vi "Generate Simulated Data.vi"(6 "Acquisition":refnum<queue>, 7 "Bits":bool[][](array[boolean]), 8 "error in (no error)":errorcluster, 10 "Longueur d'onde":dbl, 11 "Loop Count":dbl) -> (0 "error out":errorcluster, 2 "Data Out":variant[](array[variant]), 3 "Disconnected":bool=TRUE)   [LabVIEW 2018, in "Acquisition.lvlib"]
doc: "Generates sample waveforms according to the signal type in the HW Config input."
uses:
  Acquisition.lvlib
  GlobalVariable/GlobalPowerByTime.vi
  GlobalVariable/Globalt0.vi
  support/Message Queue/Message Queue.lvlib
  <vilib>/gmath/NI_Gmath.lvlib
  GlobalVariable/GlobalSet0.vi
  <vilib>/Analysis/NI_AALPro.lvlib
  GlobalVariable/GlobalPosXbyTime.vi
  GlobalVariable/GlobalPosYbyTime.vi
  GlobalVariable/GlobalProfileByTime.vi
  GlobalVariable/GlobalTimeStep.vi
  GlobalVariable/GlobalTensionByTime.vi
  GlobalVariable/GlobalTemperatureByTime.vi
  support/Message Queue/Enqueue Message (Single).vi
  <vilib>/gmath/interp.llb/Create Mesh Grid (2D) (x,y arrays).vi
  <vilib>/Analysis/2dsp.llb/2D Convolution (DBL).vi
  <vilib>/DAQmx/create/channels.llb/DAQmx Create Channel (DO-Digital Output).vi
  <resource>/objmgr/daqmx.rc
  <vilib>/Analysis/NI_AALBase.lvlib
  <vilib>/Analysis/baseanly.llb/Mean (DBL).vi
  <vilib>/DAQmx/create/channels.llb/DAQmx Create Channel (AI-Voltage-Basic).vi
  <vilib>/DAQmx/configure/timing.llb/DAQmx Timing (Sample Clock).vi
  <vilib>/DAQmx/read.llb/DAQmx Read (Analog 1D Wfm NChan NSamp).vi
  <vilib>/DAQmx/write.llb/DAQmx Write (Digital 1D Bool NChan 1Samp 1Line).vi
  support/Message Queue/Message Cluster.ctl
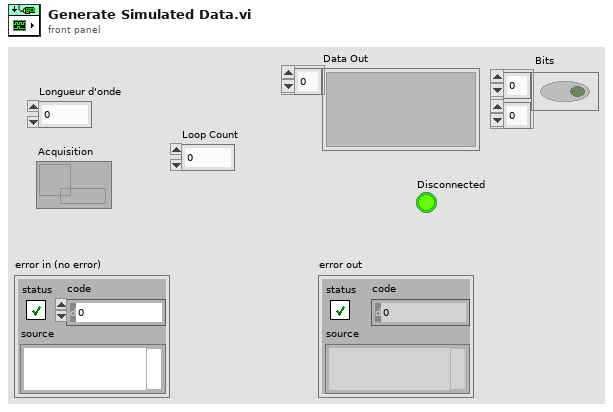
[diagram p1: front panel]
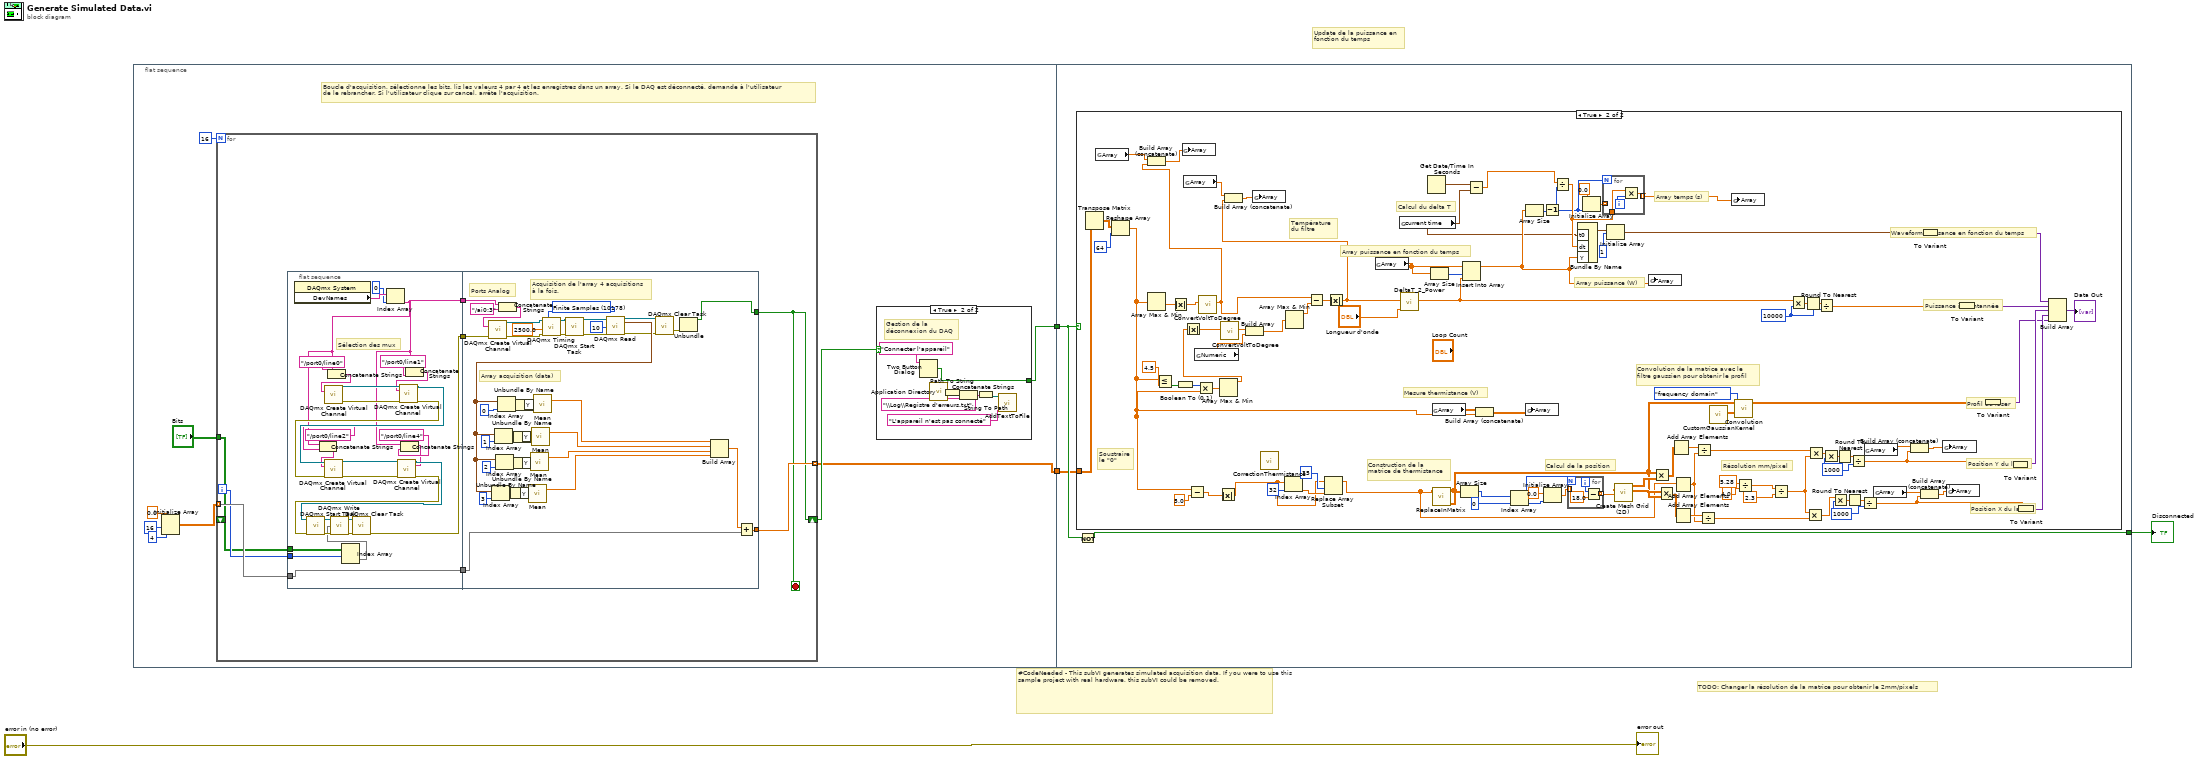
[diagram p0: block diagram]
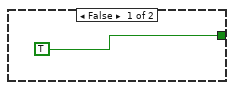
[diagram p2: hidden frame]
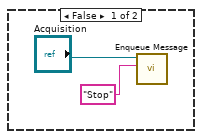
[diagram p3: hidden frame]
diagram:
  # "TODO: Changer la résolution de la matrice pour obtenir le 2mm/pixels"
  # "Update de la puissance en\nfonction du temps"
  # "#CodeNeeded - This subVI generates simulated acquisition data. If you were to use this sample project with real hardware, this subVI could be removed."
  n1 = flat-sequence {
    tunnel: [w8] -> w3
    tunnel: [w6] -> w1
    tunnel: w3 -> [w98]
    tunnel: [w97] -> w2
    tunnel: w1 -> [w96]
    frame #0 {
      # "Boucle d'acquisition, sélectionne les bits, lis les valeurs 4 par 4 et les enregistres dans un array. Si le DAQ est déconnecté, demande à l'utilisateur \nde le rebrancher. Si l'utilisateur clique sur cancel, arrête l'acquisition."
      n2 = Initialize Array(0.0 ("element"), 16 ("dimension size"), 4 ("dimension size")) -> (w9:dbl[][])
      n3 = for {
        N: 16 -> [_]
        tunnel: "Bits" -> [w25]
        tunnel: w9 -> [w30] mode=indexing
        tunnel: [w24] -> w6 mode=indexing
        shift-right: [w23] -> w7
        shift-left: _ -> [_]
        i -> [w26]
        stop <- w23 stop-if-true
        n4 = flat-sequence {
          tunnel: w26 -> [w44]
          tunnel: [w55] -> w29
          tunnel: w25 -> [w43]
          tunnel: [w31] -> w28
          tunnel: [w32] -> w27
          tunnel: w30 -> [w31]
          tunnel: w29 -> [w87]
          tunnel: w28 -> [w67]
          tunnel: [w69] -> w24
          tunnel: w27 -> [w64]
          tunnel: [w59] -> w23
          frame #0 {
            # "Sélection des mux"
            n5 = property class="DAQmx System"() -> ("DevNames"=w42:tag[])  [unwired: 2 in, 2 out]
            n6 = Index Array(array=w43, index (row)=w44) -> (element=w56:bool[])  [unwired: 1 in]
            n7 = Index Array(array=w42, index=0) -> (element=w32:tag)
            n8 = Concatenate Strings(w32, "/port0/line2" ("string")) -> (w35:string)
            n9 = Concatenate Strings(w32, "/port0/line0" ("string")) -> (w40:string)
            n10 = call-poly <vilib>:"DAQmx Create Virtual Channel.vi"("lines"=w40) -> ("task out"=w51:refnum<k21>, "error out"=w52:errorcluster)  [unwired: 13 in]
            n11 = Concatenate Strings(w32, "/port0/line4" ("string")) -> (w33:string)
            n12 = Concatenate Strings(w32, "/port0/line1" ("string")) -> (w37:string)
            n13 = call-poly <vilib>:"DAQmx Create Virtual Channel.vi"("task in"=w51, "lines"=w37, "error in"=w52) -> ("task out"=w50:refnum<k21>, "error out"=w49:errorcluster)  [unwired: 11 in]
            n14 = call-poly <vilib>:"DAQmx Create Virtual Channel.vi"("task in"=w50, "lines"=w35, "error in"=w49) -> ("task out"=w47:refnum<k21>, "error out"=w48:errorcluster)  [unwired: 11 in]
            n15 = call-poly <vilib>:"DAQmx Create Virtual Channel.vi"("task in"=w47, "lines"=w33, "error in"=w48) -> ("task out"=w46:refnum<k21>, "error out"=w45:errorcluster)  [unwired: 11 in]
            n16 = call <vilib>:"DAQmx Start Task.vi"("task/channels in"=w46, "error in"=w45) -> ("task out"=w57:refnum<k21>, "error out"=w58:errorcluster)  [unwired: 12 in]
            n17 = call-poly <vilib>:"DAQmx Write.vi"("task/channels in"=w57, "data"=w56, "error in"=w58) -> ("task out"=w54:refnum<k21>, "error out"=w53:errorcluster)  [unwired: 10 in, 1 out]
            n18 = call <vilib>:"DAQmx Clear Task.vi"("task in"=w54, "error in"=w53) -> ("error out"=w55:errorcluster)  [unwired: 13 in]
          }
          frame #1 {
            w89 = 10178 items=["Finite Samples"=10178, "Continuous Samples"=10123, "Hardware Timed Single Point"=12522] ("sample mode")
            # "Ports Analog"
            # "Array acquisition (data)"
            # "Acquisition de l'array 4 acquisitions\nà la fois."
            n19 = Concatenate Strings(w64, "/ai0:3" ("string")) -> (w65:string)
            n20 = call-poly <vilib>:"DAQmx Create Virtual Channel.vi"("physical channels"=w65, "error in"=w87) -> ("task out"=w94:refnum<k21>, "error out"=w93:errorcluster)  [unwired: 12 in]
            n21 = call-poly <vilib>:"DAQmx Timing.vi"("task/channels in"=w94, "sample mode"=w89, "rate"=2500.0, "error in"=w93) -> ("task out"=w90:refnum<k21>, "error out"=w91:errorcluster)  [unwired: 10 in]
            n22 = call <vilib>:"DAQmx Start Task.vi"("task/channels in"=w90, "error in"=w91) -> ("task out"=w92:refnum<k21>, "error out"=w95:errorcluster)  [unwired: 12 in]
            n23 = call-poly <vilib>:"DAQmx Read.vi"("task/channels in"=w92, "number of samples per channel"=10, "error in"=w95) -> ("task out"=w71:refnum<k21>, "data"=w80:waveform(dbl)[], "error out"=w70:errorcluster)  [unwired: 10 in]
            n24 = Index Array(array=w80, index=3) -> (element=w76:waveform(dbl))
            n25 = Index Array(array=w80, index=1) -> (element=w78:waveform(dbl))
            n26 = Index Array(array=w80, index=2) -> (element=w77:waveform(dbl))
            n27 = Index Array(array=w80, index=0) -> (element=w79:waveform(dbl))
            n28 = Unbundle By Name(w76) -> ("Y"=w72:dbl[])
            n29 = Unbundle By Name(w78) -> ("Y"=w74:dbl[])
            n30 = Unbundle By Name(w77) -> ("Y"=w73:dbl[])
            n31 = Unbundle By Name(w79) -> ("Y"=w75:dbl[])
            n32 = call-poly <vilib>:"Mean.vi"("X"=w72) -> ("mean"=w60:dbl)  [unwired: 1 out]
            n33 = call-poly <vilib>:"Mean.vi"("X"=w73) -> ("mean"=w61:dbl)  [unwired: 1 out]
            n34 = call-poly <vilib>:"Mean.vi"("X"=w74) -> ("mean"=w62:dbl)  [unwired: 1 out]
            n35 = call-poly <vilib>:"Mean.vi"("X"=w75) -> ("mean"=w63:dbl)  [unwired: 1 out]
            n36 = call <vilib>:"DAQmx Clear Task.vi"("task in"=w71, "error in"=w70) -> ("error out"=w85:errorcluster)  [unwired: 13 in]
            n37 = Unbundle(w85) -> ("status"=w59:bool)  [unwired: 2 out]
            n38 = Build Array(w63, w62, w61, w60) -> (w68:dbl[])
            n39 = Add(x=w68, y=w67) -> (x+y=w69:dbl[])
          }
        }
      }
      n40 = case shown="True" w7 {
        tunnel: [TRUE w22] -> w8
        frame False {
        }
        frame True {
          # "Gestion de la \ndéconnexion du DAQ"
          n41 = Two Button Dialog(message="Connecter l'appareil") -> (T button?=w22:bool)  [unwired: 2 in]
          n42 = call <vilib>:"Application Directory.vi"() -> ("Application Directory"=w19:path)
          n43 = Path To String(path=w19) -> (string=w20:string)
          n44 = Concatenate Strings(w20, "\\Log\\Registre d'erreurs.txt") -> (w21:string)
          n45 = String To Path(string=w21) -> (path=w15:path)
          n46 = call "AddTextToFile.vi"("Ajouter du texte"="L'appareil n'est pas connecté", "Fichier"=w15) -> ()  [unwired: 10 in]
        }
      }
    }
    frame #1 {
      n47 = case shown="True" w98 {
        tunnel: w96 -> [_ w101]
        frame False {
          n48 = call-poly "Enqueue Message.vi"("Message"="Stop", "Message Queue"="Acquisition") -> ()  [unwired: 8 in, 2 out]
        }
        frame True {
          w157 = 1000
          w161 = 1000
          w167 = 10000
          # "Résolution mm/pixel"
          # "Calcul du delta T"
          # "Mesure thermistance (V)"
          # "Soustraire\nle \"0\""
          # "Température \ndu filtre"
          # "Calcul de la position"
          # "Construction de la \nmatrice de thermistance"
          # "Position X du laser"
          # "Position Y du laser"
          # "Profil du laser"
          # "Puissance instantannée"
          # "Waveform puissance en fonction du temps"
          # "Array puissance (W)"
          # "Array temps (s)"
          # "Convolution de la matrice avec le \nfiltre gaussien pour obtenir le profil"
          # "Array puissance en fonction du temps"
          n49 = Transpose Matrix(1:w101) -> (0:w104:dbl[][])
          n50 = global read "GlobalTensionByTime.vi" "Array"() -> (w137:dbl[])
          n51 = Reshape Array(w104, 64 ("dimension size")) -> (w102:dbl[])
          n52 = Array Max & Min(array=w102) -> (min value=w130:dbl)  [unwired: 3 out]
          n53 = Less Or Equal?(x=w102, y=4.5) -> (x <= y?=w122:bool[])
          n54 = Absolute Value(x=w130) -> (abs(x)=w126:dbl)
          n55 = Boolean To (0,1)(Boolean=w122) -> (0, 1=w121:i16[])
          n56 = global read "GlobalTemperatureByTime.vi" "Array"() -> (w134:dbl[])
          n57 = Subtract(x=w102, y=5.0) -> (x-y=w124:dbl[])
          n58 = global read "GlobalSet0.vi" "Numeric"() -> (w108:dbl)
          n59 = Multiply(x=w121, y=w102) -> (x*y=w120:dbl[])
          n60 = call "ConvertVoltToDegree.vi"("Tension"=w126) -> ("Température"=w127:dbl)  [unwired: 10 in]
          n61 = Build Array (concatenate)(w137, w127) -> (w136:dbl[])
          n62 = global write "GlobalTensionByTime.vi" "Array"(w136) -> ()
          n63 = Array Max & Min(array=w120) -> (max value=w119:dbl)  [unwired: 3 out]
          n64 = Absolute Value(x=w119) -> (abs(x)=w128:dbl)
          n65 = Absolute Value(x=w124) -> (abs(x)=w112:dbl[])
          n66 = call "ConvertVoltToDegree.vi"("Tension"=w128) -> ("Température"=w109:dbl)  [unwired: 10 in]
          n67 = Build Array(w109, w108) -> (w106:dbl[])
          n68 = call "CorrectionThermistance.vi"() -> ()  [unwired: 11 in, 1 out]
          n69 = Index Array(array=w112, index=32) -> (element=w113:dbl)
          n70 = Array Max & Min(array=w106) -> (max value=w107:dbl)  [unwired: 3 out]
          n71 = Subtract(x=w127, y=w107) -> (x-y=w129:dbl)
          n72 = Replace Array Subset(array=w112, new element=w113, index=35) -> (w111:dbl[])
          n73 = Absolute Value(x=w129) -> (abs(x)=w116:dbl)
          n74 = Build Array (concatenate)(w134, w116) -> (w135:dbl[])
          n75 = global write "GlobalTemperatureByTime.vi" "Array"(w135) -> ()
          n76 = global read "GlobalPowerByTime.vi" "Array"() -> (w197:dbl[])
          n77 = global read "Globalt0.vi" "current time"() -> (w139:timestamp)
          n78 = call "DeltaT_2_Power.vi"("Longueur d'onde"="Longueur d'onde", "Delta T"=w116) -> ("Power"=w117:dbl)  [unwired: 9 in]
          n79 = Get Date/Time In Seconds() -> (seconds since 1Jan1904=w140:timestamp)
          n80 = Array Size(array=w197) -> (size(s)=w196:i32)
          n81 = global read "GlobalProfileByTime.vi" "Array"() -> (w143:dbl[][])
          n82 = call "ReplaceInMatrix.vi"("Input Array"=w111) -> ("Output Array"=w118:dbl[][])  [unwired: 10 in]
          n83 = Array Size(array=w118) -> (size(s)=w188:i32[])
          n84 = Insert Into Array(array=w197, index=w196, new element=w117) -> (w152:dbl[])
          n85 = Subtract(x=w140, y=w139) -> (x-y=w138:dbl)
          n86 = Build Array (concatenate)(w143, w102) -> (w144:dbl[][])
          n87 = Index Array(array=w188, index=0) -> (element=w183:i32)
          n88 = global write "GlobalProfileByTime.vi" "Array"(w144) -> ()
          n89 = Array Size(array=w152) -> (size(s)=w142:i32)
          n90 = Decrement(x=w142) -> (x-1=w141:i32)
          n91 = Initialize Array(0.0 ("element"), w183) -> (w185:dbl[])
          n92 = Divide(x=w138, y=w141) -> (x/y=w192:dbl)
          n93 = for {
            N: w183 -> [_]
            tunnel: w185 -> [_] mode=indexing
            tunnel: [w198] -> w180 mode=indexing
            i -> [w199]
            n94 = Subtract(x=w199, y=18.0) -> (x-y=w198:dbl)
          }
          n95 = Bundle By Name("t0"=w139, "dt"=w192, "Y"=w152) -> (w194:waveform(dbl))  [unwired: 1 in]
          n96 = Initialize Array(0.0 ("element"), w141) -> (w190:dbl[])
          n97 = for {
            N: w141 -> [_]
            tunnel: w192 -> [w202]
            tunnel: w190 -> [_] mode=indexing
            tunnel: [w201] -> w151 mode=indexing
            i -> [w203]
            n98 = Multiply(x=w202, y=w203) -> (x*y=w201:dbl)
          }
          n99 = Initialize Array(w194, 1) -> (w171:waveform(dbl)[])
          n100 = call-poly <vilib>:"Create Mesh Grid (2D).vi"("y domain"=w180, "x domain"=w180) -> ("Y"=w179:dbl[][], "X"=w184:dbl[][])  [unwired: 7 in, 1 out]
          n101 = global write "GlobalPowerByTime.vi" "Array"(w152) -> ()
          n102 = Multiply(x=w118, y=w184) -> (x*y=w182:dbl[][])
          n103 = Multiply(x=w179, y=w118) -> (x*y=w178:dbl[][])
          n104 = Add Array Elements(numeric array=w182) -> (sum=w181:dbl)
          n105 = Add Array Elements(numeric array=w111) -> (sum=w176:dbl)
          n106 = Add Array Elements(numeric array=w178) -> (sum=w177:dbl)
          n107 = Divide(x=w181, y=w176) -> (x/y=w174:dbl)
          n108 = Divide(x=w177, y=w176) -> (x/y=w175:dbl)
          n109 = call "CustomGaussianKernel.vi"() -> ("array"=w189:dbl[][])  [unwired: 11 in]
          n110 = global write "GlobalTimeStep.vi" "Array"(w151) -> ()
          n111 = call-poly <vilib>:"Convolution.vi"("algorithm"=enum32{"direct", "frequency domain"}."frequency domain", "Y"=w189, "X"=w118) -> ("X * Y"=w131:dbl[][])  [unwired: 7 in, 1 out]
          n112 = Divide(x=5.28, y=4.0) -> (x/y=w133:dbl)
          n113 = Divide(x=w133, y=2.3) -> (x/y=w132:dbl)
          n114 = Multiply(x=w117, y=w167) -> (x*y=w168:dbl)
          n115 = Round To Nearest(number=w168) -> (nearest integer value=w166:dbl)
          n116 = Multiply(x=w132, y=w175) -> (x*y=w154:dbl)
          n117 = Multiply(x=w174, y=w132) -> (x*y=w158:dbl)
          n118 = Divide(x=w166, y=w167) -> (x/y=w162:dbl)
          n119 = Multiply(x=w158, y=w161) -> (x*y=w160:dbl)
          n120 = Multiply(x=w154, y=w157) -> (x*y=w156:dbl)
          n121 = Round To Nearest(number=w160) -> (nearest integer value=w159:dbl)
          n122 = Round To Nearest(number=w156) -> (nearest integer value=w155:dbl)
          n123 = Divide(x=w159, y=w161) -> (x/y=w145:dbl)
          n124 = Divide(x=w155, y=w157) -> (x/y=w149:dbl)
          n125 = global read "GlobalPosXbyTime.vi" "Array"() -> (w146:dbl[])
          n126 = global read "GlobalPosYbyTime.vi" "Array"() -> (w150:dbl[])
          n127 = Build Array (concatenate)(w146, w145) -> (w147:dbl[])
          n128 = Build Array (concatenate)(w150, w149) -> (w148:dbl[])
          n129 = To Variant(anything=w171) -> (Variant=w170:variant)
          n130 = global write "GlobalPosXbyTime.vi" "Array"(w147) -> ()
          n131 = global write "GlobalPosYbyTime.vi" "Array"(w148) -> ()
          n132 = To Variant(anything=w162) -> (Variant=w163:variant)
          n133 = To Variant(anything=w131) -> (Variant=w153:variant)
          n134 = To Variant(anything=w145) -> (Variant=w164:variant)
          n135 = To Variant(anything=w149) -> (Variant=w165:variant)
          n136 = Build Array(w170, w163, w164, w165, w153) -> (→"Data Out":variant[])
        }
      }
      n137 = Not(x=w98) -> (.not. x?=w97:bool)
    }
  }
  "error out" <- "error in (no error)"
  "Disconnected" <- w2
